vi "get_mode.vi"(8 "error in":errorcluster, 11 "VISA resource name":refnum<visa-resource-name>="COM1") -> (0 "error out":errorcluster, 3 "VISA resource name out":refnum<visa-resource-name>)   [LabVIEW 2020]
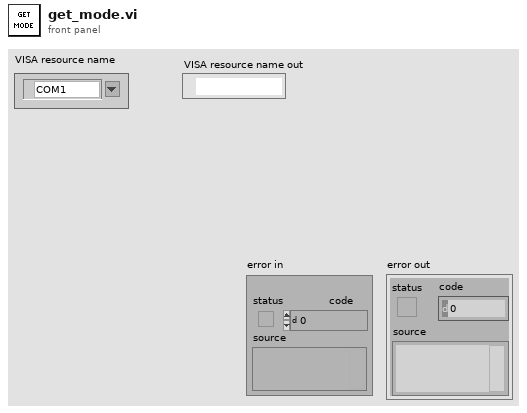
[diagram p1: front panel]
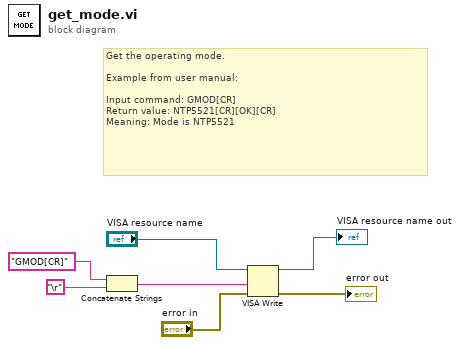
[diagram p0: block diagram]
diagram:
  # "Get the operating mode.\n\nExample from user manual:\n\nInput command: GMOD[CR]\nReturn value: NTP5521[CR][OK][CR]\nMeaning: Mode is NTP5521"
  n1 = Concatenate Strings("GMOD[CR]" ("Command"), "\r") -> (w4:string)
  n2 = VISA Write(VISA resource name="VISA resource name", write buffer=w4, error in (no error)="error in") -> (VISA resource name out=→"VISA resource name out":refnum<visa-resource-name>, error out=→"error out":errorcluster)  [unwired: 1 out]
